vi "SetWatchdogTimer.vi"(8 "error in":errorcluster, 10 "Watchdog timer seconds (0-600)":i16 min=0 max=600 step=1, 11 "VISA resource name":refnum<visa-resource-name>) -> (0 "error out":errorcluster, 2 "Reset watchdog timer result":string, 3 "VISA resource name out":refnum<visa-resource-name>)   [LabVIEW 2023, in "Thermotron 8800.lvlib"]
doc: "WDOG\nCommand name: Reset watchdog timer\nCommand type: Control\nDescription: This command provides an extra level of protection for users operating their chambers entirely through the computer interface. The watchdog operates as a “everything is OK” command. If the watchdog is enabled and happens to time out due to a loss of communication, the controller will enter a known fail-safe state by running a program called failsafe.pgm. If that particular program does not exist, the chamber will simply enter the stop mode. The syntax for the command is WDOGn, where n is a number of seconds between 0 and 600. A positive value sets the watchdog timer value. A zero value turns off the watchdog feature. Once the watchdog is set, the 8800 internally begins counting down. If the internal watchdog timer ever reaches 0, the 8800 will enter the fail-safe state. For this reason you must periodically send the WDOGn command to reset the watchdog timer.\nSyntax: WDOGn\nWhere n is the number of seconds between 0 and 600.\nData type: No data\nOperation example: WDOG30\n8800 response: The 8800 resets the internal watchdog timer to 30 seconds."
uses:
  Thermotron 8800.lvlib
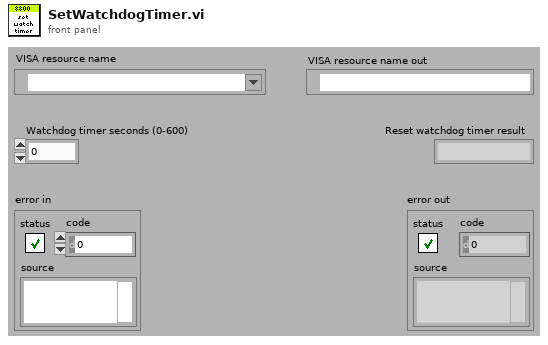
[diagram p1: front panel]
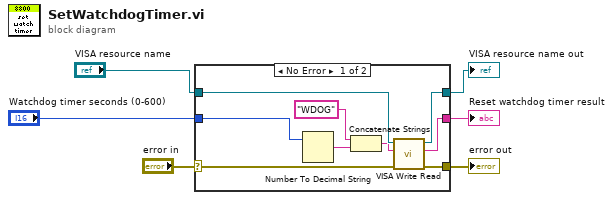
[diagram p0: block diagram]
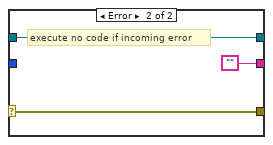
[diagram p2: hidden frame]
diagram:
  n1 = case shown="No Error" "error in" {
    selector: "error in" -> [w12 w18]
    tunnel: "VISA resource name" -> [w15 w17]
    tunnel: [w14 w17] -> w5
    tunnel: [w13 w18] -> w4
    tunnel: [w11 ""] -> w2
    tunnel: "Watchdog timer seconds (0-600)" -> [w7 _]
    frame No Error {
      n2 = Number To Decimal String(number=w7) -> (decimal integer string=w8:string)  [unwired: 1 in]
      n3 = Concatenate Strings("WDOG" ("8800 Command"), w8) -> (w9:string)
      n4 = call "VISA Write Read.vi"("error in (no error)"=w12, "8800 Command"=w9, "VISA Refnum in"=w15) -> ("error out"=w13:errorcluster, "read buffer"=w11:string, "VISA Refnum out"=w14:refnum<visa-resource-name>)  [unwired: 6 in]
    }
    frame Error {
      # "execute no code if incoming error"
    }
  }
  "VISA resource name out" <- w5
  "error out" <- w4
  "Reset watchdog timer result" <- w2
